vi "Begin.vi"   [LabVIEW 2012]
doc: "Called before other user functions, this VI is expected to open initial I/O refnums, load in file data, and do all program initialization. Notice that the <B>error out</B> terminal is simply used for data flow. Wiring it to other structures or subVIs ensures that this VI runs first."
uses:
  <vilib>/Rock Robotics/WPI/DriverStation/WPI_DriverStationRobotMode2.ctl
  <vilib>/Rock Robotics/WPI/CAN/Jaguar/SubVIs/WPI_CANJaguar_ControlMode.ctl
  <vilib>/Rock Robotics/WPI/CAN/Jaguar/SubVIs/WPI_CANJaguar_SpeedReference.ctl
  <vilib>/Rock Robotics/WPI/Joystick/WPI_JoystickDeviceEnum.ctl
  Robot Global Data.vi
  <vilib>/Rock Robotics/WPI/MotorControl/WPI_MotorControlOpenCANJaguar.vi
types:
  T1 = typedef "WPI_JoystickDeviceEnum.ctl" = enum16{"USB 1", "USB 2", "USB 3", "USB 4", "Kinect 1", "Kinect 2"}
  T2 = typedef "WPI_CANJaguar_SpeedReference.ctl" = u8
  T3 = typedef "WPI_CANJaguar_ControlMode.ctl" = enum8{"Percent VBus", "Current", "Speed", "Position", "Voltage"}
  T4 = typedef "WPI_DriverStationRobotMode2.ctl" = enum16{"Autonomous Disabled", "Autonomous Enabled", "Teleop Disabled", "Teleop Enabled", "Timeout", "Finish", "Test Disabled", "Test Enabled"}
  T5 = typedef "WPI_JoystickDevRef.ctl" = cluster{"Device":T1}
  T6 = typedef "WPI_MotorControlDeviceRef.ctl" = cluster{"DeviceStatus":errorcluster, "Type":enum16{"PWM", "CAN"}, "PWM":cluster{"Digital Module":T7, "PWM Channel":T8, "DeadBand":T9}, "CAN":cluster{"Device Number":u8, "Control Mode":T3, "Semaphore":T10, "Max Vout":dbl}, "Invert":bool, "TransformRef":T11, "InvTransformRef":T11}
  T7 = typedef "FPGA_TypedefDigitalModule.ctl" = enum16{"Digital Module 1", "Digital Module 2"}
  T8 = typedef "FPGA_DIOPWMChannel.ctl" = enum8{"PWM 1", "PWM 2", "PWM 3", "PWM 4", "PWM 5", "PWM 6", "PWM 7", "PWM 8", "PWM 9", "PWM 10", "Invalid"}
  T9 = typedef "WPI_PWMDeadband.ctl" = cluster{"Name":string, "maxPositivePwm":i32, "minPositivePwm":i32, "centerPwm":i32, "maxNegativePwm":i32, "minNegativePwm":i32, "angularRange":u16}
  T10 = typedef "Semaphore RefNum" = refnum<k1>
  T11 = typedef "WPI_PWMTransform_ConPane.ctl" = refnum<vi>
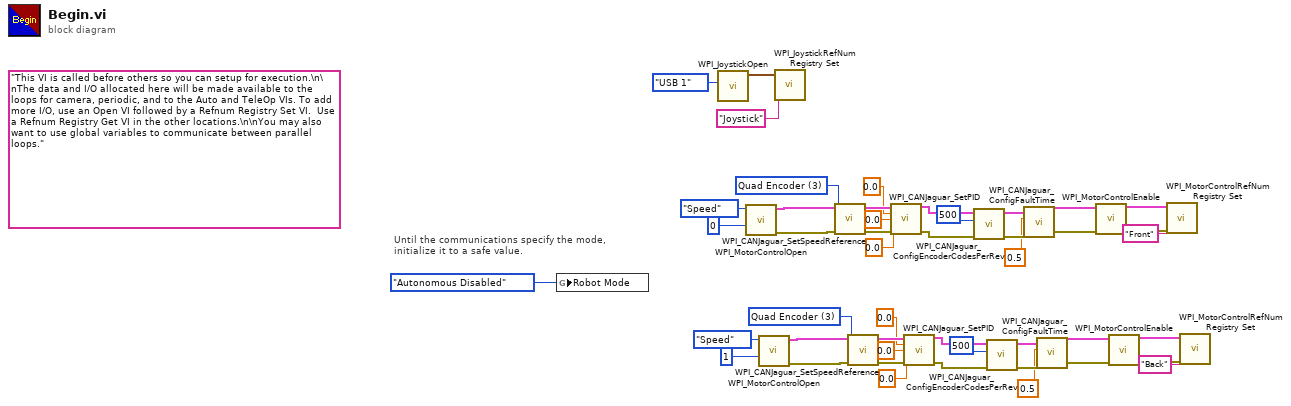
[diagram p0: block diagram]
diagram:
  w23 = T2 3 items=["Encoder"=0, "Inv Encoder"=2, "Quad Encoder"=3, "None"=255] ("Speed Reference")
  w43 = T2 3 items=["Encoder"=0, "Inv Encoder"=2, "Quad Encoder"=3, "None"=255] ("Speed Reference")
  (unwired) "This VI is called before others so you can setup for execution.\n\nThe data and I/O allocated here will be made available to the loops for camera, periodic, and to the Auto and TeleOp VIs. To add more I/O, use an Open VI followed by a Refnum Registry Set VI.  Use a Refnum Registry Get VI in the other locations.\n\nYou may also want to use global variables to communicate between parallel loops."
  # "Until the communications specify the mode,\ninitialize it to a safe value."
  n1 = global write "Robot Global Data.vi" "Robot Mode"(WPI_DriverStationRobotMode2."Autonomous Disabled" ("Robot Mode")) -> ()
  n2 = call <vilib>:"WPI_JoystickOpen.vi"("JoystickDevice"=WPI_JoystickDeviceEnum."USB 1") -> ("JoystickDevRef"=w2:T5)  [unwired: 10 in]
  n3 = call-poly <vilib>:"WPI_MotorControlOpen.vi"("Device Number"=u8 0, "Control Mode"=WPI_CANJaguar_ControlMode."Speed") -> ("error out"=w21:errorcluster, "MotorControlDeviceRef"=w22:T6)  [unwired: 8 in]
  n4 = call-poly <vilib>:"WPI_MotorControlOpen.vi"("Device Number"=u8 1, "Control Mode"=WPI_CANJaguar_ControlMode."Speed") -> ("error out"=w41:errorcluster, "MotorControlDeviceRef"=w42:T6)  [unwired: 8 in]
  n5 = call <vilib>:"WPI_JoystickRefNum Registry Set.vi"("refnum name"="Joystick", "JoystickDevRef"=w2) -> ()  [unwired: 8 in, 2 out]
  n6 = call <vilib>:"WPI_CANJaguar_SetSpeedReference.vi"("error in (no error)"=w21, "Speed Reference"=w23, "CAN Jaguar Ref"=w22) -> ("error out"=w19:errorcluster, "CAN Jaguar Ref Out"=w20:T6)  [unwired: 7 in]
  n7 = call <vilib>:"WPI_CANJaguar_SetSpeedReference.vi"("error in (no error)"=w41, "Speed Reference"=w43, "CAN Jaguar Ref"=w42) -> ("error out"=w39:errorcluster, "CAN Jaguar Ref Out"=w40:T6)  [unwired: 7 in]
  n8 = call <vilib>:"WPI_CANJaguar_SetPID.vi"("CAN Jaguar Ref"=w20, "P"=0.0, "I"=0.0, "D"=0.0, "error in (no error)"=w19) -> ("CAN Jaguar Ref Out"=w14:T6, "error out"=w15:errorcluster)  [unwired: 9 in]
  n9 = call <vilib>:"WPI_CANJaguar_SetPID.vi"("CAN Jaguar Ref"=w40, "P"=0.0, "I"=0.0, "D"=0.0, "error in (no error)"=w39) -> ("CAN Jaguar Ref Out"=w34:T6, "error out"=w35:errorcluster)  [unwired: 9 in]
  n10 = call <vilib>:"WPI_CANJaguar_ConfigEncoderCodesPerRev.vi"("error in (no error)"=w15, "Encoder Codes Per Rev"=u16 500, "CAN Jaguar Ref"=w14) -> ("error out"=w12:errorcluster, "CAN Jaguar Ref Out"=w11:T6)  [unwired: 7 in]
  n11 = call <vilib>:"WPI_CANJaguar_ConfigEncoderCodesPerRev.vi"("error in (no error)"=w35, "Encoder Codes Per Rev"=u16 500, "CAN Jaguar Ref"=w34) -> ("error out"=w32:errorcluster, "CAN Jaguar Ref Out"=w31:T6)  [unwired: 7 in]
  n12 = call <vilib>:"WPI_CANJaguar_ConfigFaultTime.vi"("error in (no error)"=w12, "Fault Time (s)"=0.5, "CAN Jaguar Ref"=w11) -> ("error out"=w8:errorcluster, "CAN Jaguar Ref Out"=w9:T6)  [unwired: 7 in]
  n13 = call <vilib>:"WPI_CANJaguar_ConfigFaultTime.vi"("error in (no error)"=w32, "Fault Time (s)"=0.5, "CAN Jaguar Ref"=w31) -> ("error out"=w28:errorcluster, "CAN Jaguar Ref Out"=w29:T6)  [unwired: 7 in]
  n14 = call <vilib>:"WPI_MotorControlEnable.vi"("error in (no error)"=w8, "CAN Jaguar Ref"=w9) -> ("error out"=w6:errorcluster, "CAN Jaguar Ref Out"=w7:T6)  [unwired: 8 in]
  n15 = call <vilib>:"WPI_MotorControlEnable.vi"("error in (no error)"=w28, "CAN Jaguar Ref"=w29) -> ("error out"=w26:errorcluster, "CAN Jaguar Ref Out"=w27:T6)  [unwired: 8 in]
  n16 = call <vilib>:"WPI_MotorControlRefNum Registry Set.vi"("error in (no error)"=w6, "refnum name"="Front", "MotorControlDevRef"=w7) -> ()  [unwired: 7 in, 2 out]
  n17 = call <vilib>:"WPI_MotorControlRefNum Registry Set.vi"("error in (no error)"=w26, "refnum name"="Back", "MotorControlDevRef"=w27) -> ()  [unwired: 7 in, 2 out]
